vi "индикатор.vi"() -> ()   [LabVIEW 2019]
panel:
  in  "Ring":u16(ring) items=["0", "1", "2", "3", "4", "5", "6", "7", "8", "9"]
  in  "stop":bool
  out "Boolean 7":bool
  out "Boolean 6":bool
  out "Boolean 5":bool
  out "Boolean 4":bool
  out "Boolean 3":bool
  out "Boolean 2":bool
  out "Boolean":bool
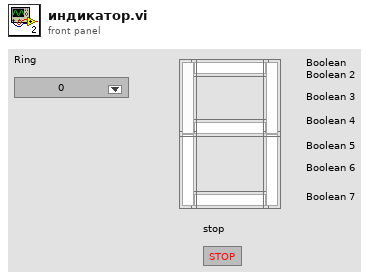
[diagram p1: front panel]
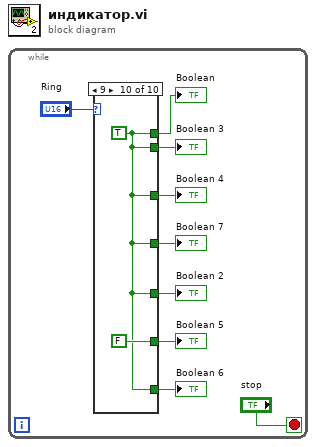
[diagram p0: block diagram]
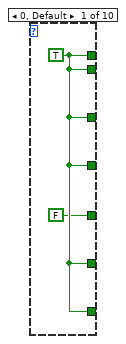
[diagram p2: hidden frame]
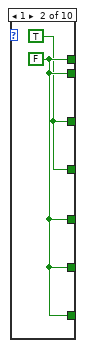
[diagram p3: hidden frame]
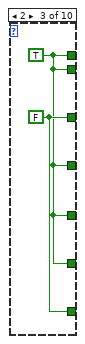
[diagram p4: hidden frame]
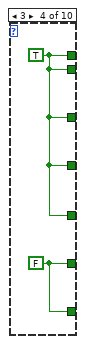
[diagram p5: hidden frame]
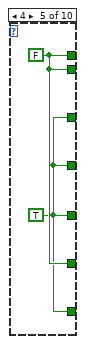
[diagram p6: hidden frame]
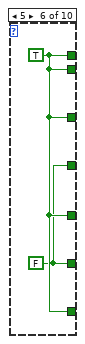
[diagram p7: hidden frame]
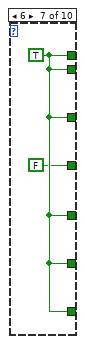
[diagram p8: hidden frame]
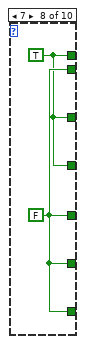
[diagram p9: hidden frame]
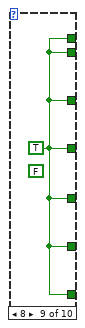
[diagram p10: hidden frame]
diagram:
  n1 = while {
    stop <- "stop" stop-if-true
    n2 = case shown="9" "Ring" {
      tunnel: [w11 w13 w14 w16 w19 w21 w23 w24 w26 w27] -> w7
      tunnel: [FALSE w13 w14 w16 w18 w21 w23 w25 w26 w27] -> w6
      tunnel: [w11 w13 w14 w16 w19 w21 w23 w25 w26 w27] -> w5
      tunnel: [w11 w12 w15 w16 w18 w21 w23 w24 w26 w27] -> w4
      tunnel: [w11 w13 w14 w17 w19 w20 w23 w25 w26 FALSE] -> w3
      tunnel: [w11 w13 w15 w17 w18 w21 w23 w25 w26 w27] -> w2
      tunnel: [w11 w12 w14 w16 w18 w20 FALSE w24 w26 w27] -> w1
      frame 0, Default {
        w11 = TRUE
      }
      frame 1 {
        w13 = FALSE
        w12 = TRUE
      }
      frame 2 {
        w15 = FALSE
        w14 = TRUE
      }
      frame 3 {
        w17 = FALSE
        w16 = TRUE
      }
      frame 4 {
        w19 = FALSE
        w18 = TRUE
      }
      frame 5 {
        w20 = FALSE
        w21 = TRUE
      }
      frame 6 {
        w23 = TRUE
      }
      frame 7 {
        w25 = FALSE
        w24 = TRUE
      }
      frame 8 {
        (unwired) FALSE
        w26 = TRUE
      }
      frame 9 {
        w27 = TRUE
      }
    }
    "Boolean" <- w7
    "Boolean 2" <- w6
    "Boolean 3" <- w5
    "Boolean 4" <- w4
    "Boolean 5" <- w3
    "Boolean 6" <- w2
    "Boolean 7" <- w1
  }
